vi "Joystick - Logitech Attack 3 - Right - Get All.vi"(8 "error in (no error)":errorcluster) -> (0 "error out":errorcluster, 2 "Buttons [Cluster]":T1={"Trigger Button 1"=TRUE, "Thumb Button 2 "=TRUE, "Thumb Button 3"=TRUE, "Thumb Button 4"=TRUE, "Thumb Button 5"=TRUE, "Bottom Button 6"=TRUE, "Bottom Button 7"=TRUE, "Bottom Button 8"=TRUE, "Bottom Button 9"=TRUE, "Bottom Button 10"=TRUE, "Bottom Button 11"=TRUE}, 3 "Axes [Cluster]":T2, 4 "Buttons":bool[](array[boolean]), 6 "Axes":dbl[](array[numeric]))   [LabVIEW 2015]
uses:
  Logitech Attack 3 Axis Map.ctl
  Logitech Attack 3 Button Map.ctl
  <vilib>/Rock Robotics/WPI/Utilities/WPI_GetSetVariantRefNum.vi
  <vilib>/Rock Robotics/Network Tables/NT Write Numeric Array.vi
  <vilib>/Rock Robotics/Network Tables/NT Write Boolean Array.vi
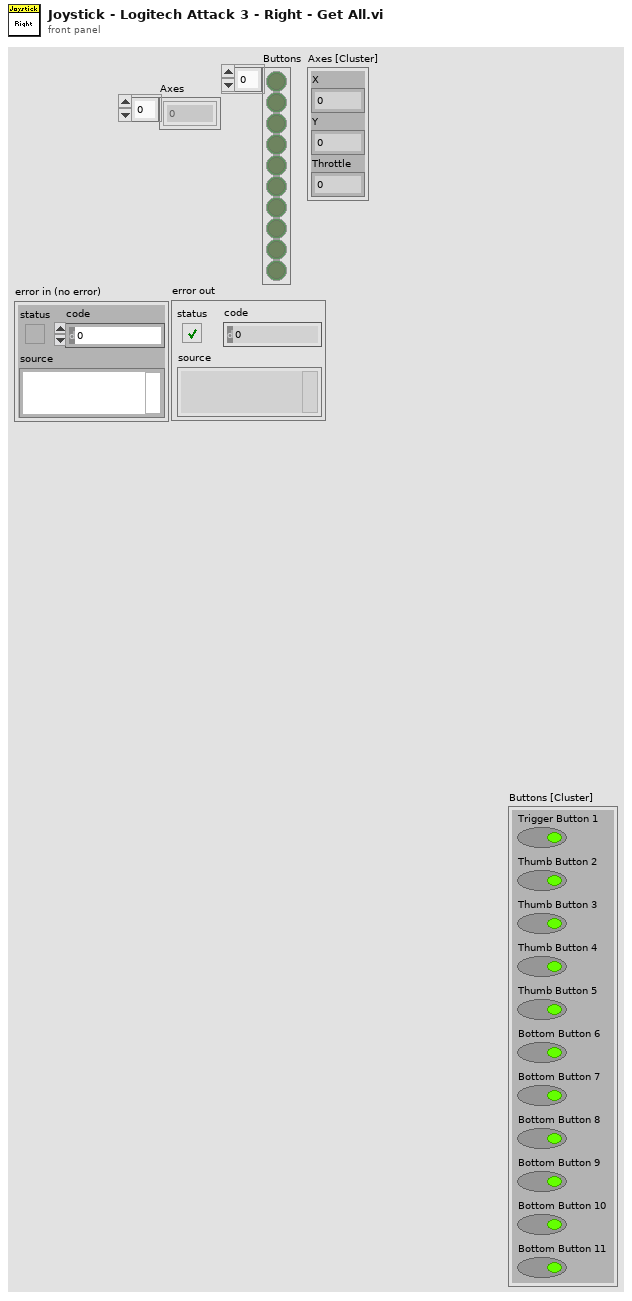
[diagram p1: front panel]
types:
  T1 = typedef "Logitech Attack 3 Button Map.ctl" = cluster{"Trigger Button 1":bool, "Thumb Button 2 ":bool, "Thumb Button 3":bool, "Thumb Button 4":bool, "Thumb Button 5":bool, "Bottom Button 6":bool, "Bottom Button 7":bool, "Bottom Button 8":bool, "Bottom Button 9":bool, "Bottom Button 10":bool, "Bottom Button 11":bool}
  T2 = typedef "Logitech Attack 3 Axis Map.ctl" = cluster{"X":dbl, "Y":dbl, "Throttle":dbl}
  T3 = typedef "WPI_JoystickDevRef.ctl" = cluster{"Device":T4}
  T4 = typedef "WPI_JoystickDeviceEnum.ctl" = enum16{"USB 0", "USB 1", "USB 2", "USB 3", "USB 4", "USB 5"}
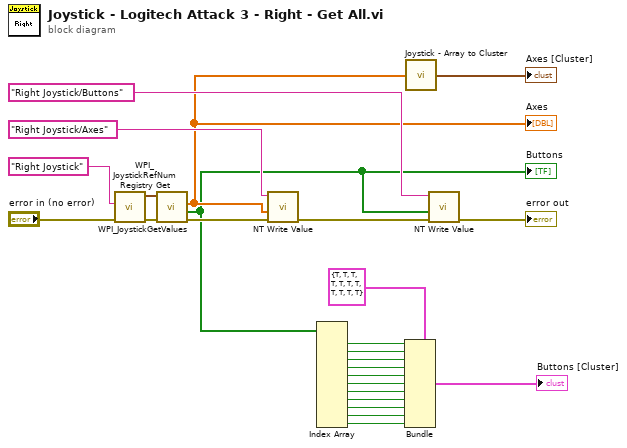
[diagram p0: block diagram]
diagram:
  n1 = call <vilib>:"WPI_JoystickRefNum Registry Get.vi"("error in (no error)"="error in (no error)", "refnum name"="Right Joystick") -> ("error out"=w21:errorcluster, "JoystickDevRef"=w22:T3)  [unwired: 8 out]
  n2 = call <vilib>:"WPI_JoystickGetValues.vi"("error in (no error)"=w21, "JoystickDevRef"=w22) -> ("error out"=w20:errorcluster, "Buttons"=w1:bool[], "Axes"=w15:dbl[])  [unwired: 5 in, 2 out]
  "Axes" <- w15
  "Buttons" <- w1
  n3 = call-poly <vilib>:"NT Write Value.vi"("error in"=w20, "Numeric Array"=w15, "Name"="Right Joystick/Axes") -> ("error out"=w19:errorcluster)  [unwired: 8 in]
  n4 = Index Array(array=w1) -> (element #1=w13:bool, element #2=w12:bool, element #3=w11:bool, element #4=w10:bool, element #5=w9:bool, element #6=w8:bool, element #7=w6:bool, element #8=w7:bool, element #9=w5:bool, element #10=w4:bool, element #11=w3:bool)  [unwired: 11 in]
  n5 = Bundle(cluster=T1 {"Trigger Button 1"=TRUE, "Thumb Button 2 "=TRUE, "Thumb Button 3"=TRUE, "Thumb Button 4"=TRUE, "Thumb Button 5"=TRUE, "Bottom Button 6"=TRUE, "Bottom Button 7"=TRUE, "Bottom Button 8"=TRUE, "Bottom Button 9"=TRUE, "Bottom Button 10"=TRUE, "Bottom Button 11"=TRUE}, "Trigger Button 1"=w13, "Thumb Button 2"=w12, "Thumb Button 3"=w11, "Thumb Button 4"=w10, "Thumb Button 5"=w9, "Bottom Button 6"=w8, "Bottom Button 7"=w6, "Bottom Button 8"=w7, "Bottom Button 9"=w5, "Bottom Button 10"=w4, "Bottom Button 11"=w3) -> (→"Buttons [Cluster]":T1)
  n6 = call "Joystick - Array to Cluster.vi"("Axes"=w15) -> ("Axes [Cluster]"=→"Axes [Cluster]":T2)
  n7 = call-poly <vilib>:"NT Write Value.vi"("error in"=w19, "Boolean Array"=w1, "Name"="Right Joystick/Buttons") -> ("error out"=→"error out":errorcluster)  [unwired: 8 in]
